vi "circle.vi"() -> ()   [LabVIEW 2023]
doc: "A VI with a moving cirle graph."
panel:
  in  "stop":bool
  in  "radius":dbl min=0.0
  out "XY Graph":cluster{"X":dbl, "Y":dbl}[](graph)
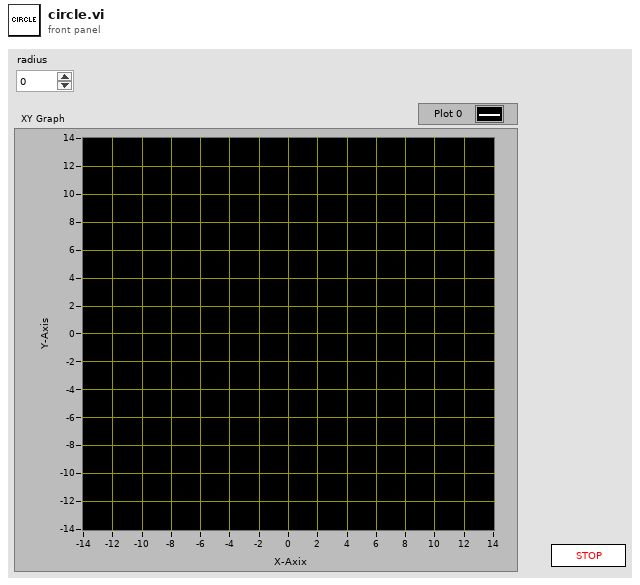
[diagram p1: front panel]
types:
  T1 = cluster{"radius":dbl, "x_offset":dbl, "y_offset":dbl}
  T2 = typedef "eventvkey.ctl" = enum16{"ASCII", "Enter", "Return", "Shift", "Ctrl", "Alt", "Cmd", "Opt", "Caps", "NumLock", "Clear", "Break", "Up", "Down", "Left", "Right", "Insert", "Delete", "Home", "End", "PageUp", "PageDown", "Escape", "Help", "Pause", "ScrollLock", "F1", "F2", "F3", "F4", "F5", "F6", "F7", "F8", "F9", "F10", "F11", "F12", "F13", "F14", "F15", "F16", "F17", "F18", "F19", "F20", "F21", "F22", "F23", "F24", "Play", "VolumeUp", "VolumeDown", "Mute", "Two Byte Char"}
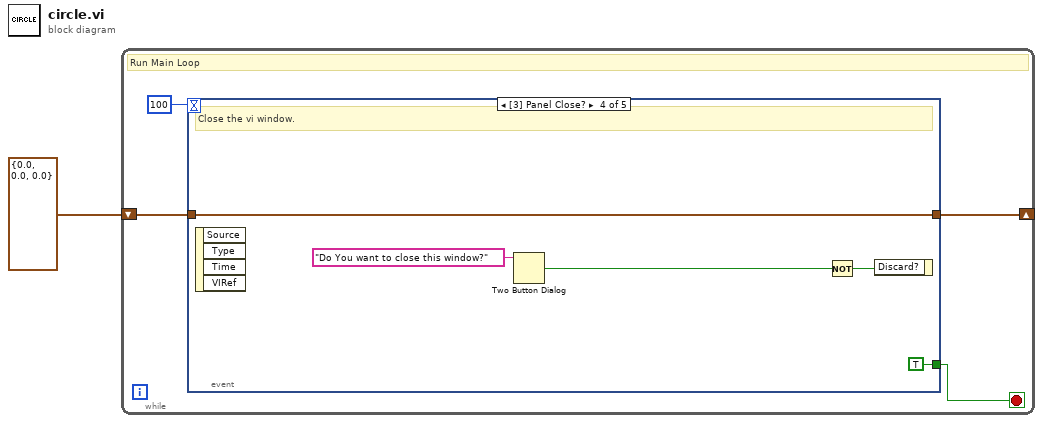
[diagram p0: block diagram]
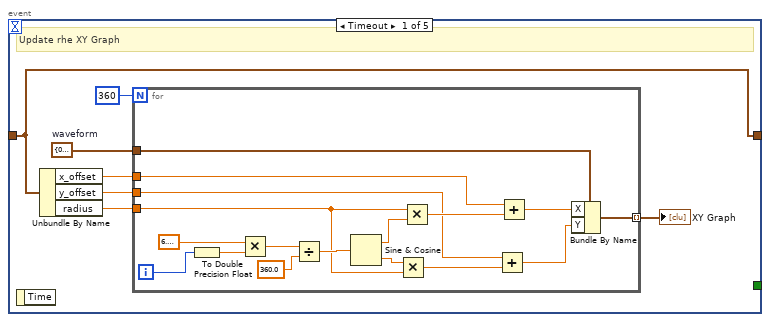
[diagram p2: hidden frame]
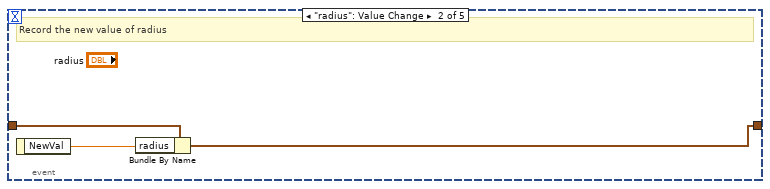
[diagram p3: hidden frame]
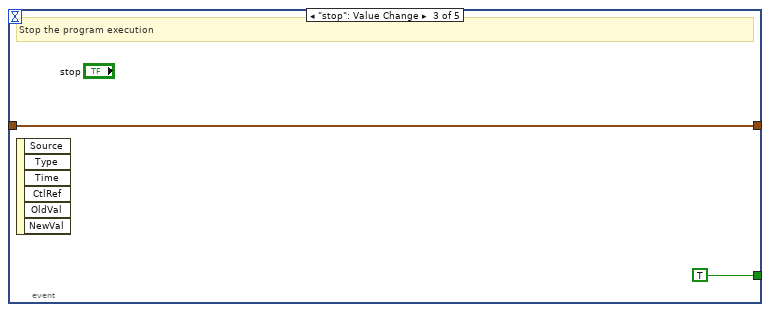
[diagram p4: hidden frame]
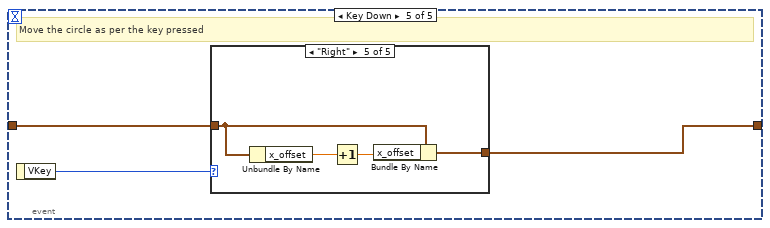
[diagram p5: hidden frame]
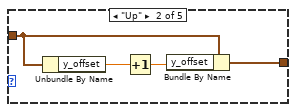
[diagram p7: hidden frame]
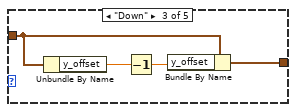
[diagram p8: hidden frame]
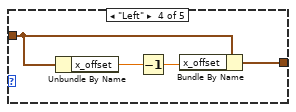
[diagram p9: hidden frame]
diagram:
  n1 = while {
    shift-right: [w3] -> _
    shift-left: T1 {"radius"=0.0, "x_offset"=0.0, "y_offset"=0.0} -> [w4]
    stop <- w2 stop-if-true
    # "Run Main Loop"
    n2 = event shown="[3] Panel Close?" {
      selector: _ -> [_ _ _ _ _]
      dyn-events: _ -> [_ _ _ _ _]
      timeout: 100 -> [_ _ _ _ _]
      tunnel: w4 -> [w10 w32 w34 w39 w41]
      tunnel: [w10 w31 w34 w39 w40] -> w3
      tunnel: [_ _ TRUE TRUE _] -> w2
      event Timeout {
        w11 = cluster{"X":dbl, "Y":dbl} {"X"=0.0, "Y"=0.0}  # waveform
        # "Update rhe XY Graph"
        n3 = event-data() -> ()  [unwired: 1 in, 1 out]
        n4 = Unbundle By Name(w10) -> ("x_offset"=w7:dbl, "y_offset"=w6:dbl, "radius"=w9:dbl)
        n5 = for {
          N: 360 -> [_]
          tunnel: [w23] -> w8 mode=indexing
          tunnel: w9 -> [w18]
          tunnel: w11 -> [w20]
          tunnel: w7 -> [w14]
          tunnel: w6 -> [w13]
          i -> [w29]
          n6 = To Double Precision Float(number=w29) -> (double precision float=w27:dbl)
          n7 = Multiply(x=6.283185307179586, y=w27) -> (x*y=w26:dbl)
          n8 = Divide(x=w26, y=360.0) -> (x/y=w24:dbl)
          n9 = Sine & Cosine(0:w24) -> (1:w19:dbl, 2:w22:dbl)
          n10 = Multiply(x=w22, y=w18) -> (x*y=w15:dbl)
          n11 = Multiply(x=w18, y=w19) -> (x*y=w21:dbl)
          n12 = Add(x=w13, y=w15) -> (x+y=w16:dbl)
          n13 = Add(x=w14, y=w21) -> (x+y=w17:dbl)
          n14 = Bundle By Name(cluster=w20, "X"=w17, "Y"=w16) -> (w23:cluster{"X":dbl, "Y":dbl})
        }
        "XY Graph" <- w8
      }
      event "radius": Value Change {
        # "Record the new value of radius"
        n15 = event-data() -> ("NewVal"=w30:dbl)  [unwired: 1 in]
        n16 = Bundle By Name(cluster=w32, "radius"=w30) -> (w31:T1)
      }
      event "stop": Value Change {
        # "Stop the program execution"
        n17 = event-data() -> ()  [unwired: 1 in, 6 out]
      }
      event Panel Close? {
        # "Close the vi window."
        n18 = event-data() -> ()  [unwired: 1 in, 4 out]
        n19 = Two Button Dialog(message="Do You want to close this window?") -> (T button?=w36:bool)  [unwired: 2 in]
        n20 = Not(x=w36) -> (.not. x?=w37:bool)
        n21 = event-data("Discard?"=w37) -> ()  [unwired: 1 in, 1 out]
      }
      event Key Down {
        # "Move the circle as per the key pressed"
        n22 = event-data() -> ("VKey"=w42:T2)  [unwired: 1 in]
        n23 = case shown="\"Right\"" w42 {
          tunnel: w41 -> [w43 w45 w49 w53 w59]
          tunnel: [w43 w44 w48 w52 w56] -> w40
          frame "ASCII", Default {
          }
          frame "Up" {
            n24 = Unbundle By Name(w45) -> ("y_offset"=w46:dbl)
            n25 = Increment(x=w46) -> (x+1=w47:dbl)
            n26 = Bundle By Name(cluster=w45, "y_offset"=w47) -> (w44:T1)
          }
          frame "Down" {
            n27 = Unbundle By Name(w49) -> ("y_offset"=w50:dbl)
            n28 = Decrement(x=w50) -> (x-1=w51:dbl)
            n29 = Bundle By Name(cluster=w49, "y_offset"=w51) -> (w48:T1)
          }
          frame "Left" {
            n30 = Unbundle By Name(w53) -> ("x_offset"=w54:dbl)
            n31 = Decrement(x=w54) -> (x-1=w55:dbl)
            n32 = Bundle By Name(cluster=w53, "x_offset"=w55) -> (w52:T1)
          }
          frame "Right" {
            n33 = Unbundle By Name(w59) -> ("x_offset"=w57:dbl)
            n34 = Increment(x=w57) -> (x+1=w58:dbl)
            n35 = Bundle By Name(cluster=w59, "x_offset"=w58) -> (w56:T1)
          }
        }
      }
    }
  }
